vi "MODEL SELECTION.vi"(8 "error in (no error)":errorcluster, 11 "Plan List":string[](array[string])) -> (0 "error out 2":errorcluster, 2 "SELECTED RECIPE\nand COMBI OF BIN- INDEX":cluster{"RECIPE INDEX":i32, "COMBI BIN":i32}, 3 "Plan Selected":string(combo))   [LabVIEW 2017]
panel:
  in  "RECIPE SELECT":string(combo)
  in  "Cancel Button":bool
  in  "Save Button":bool
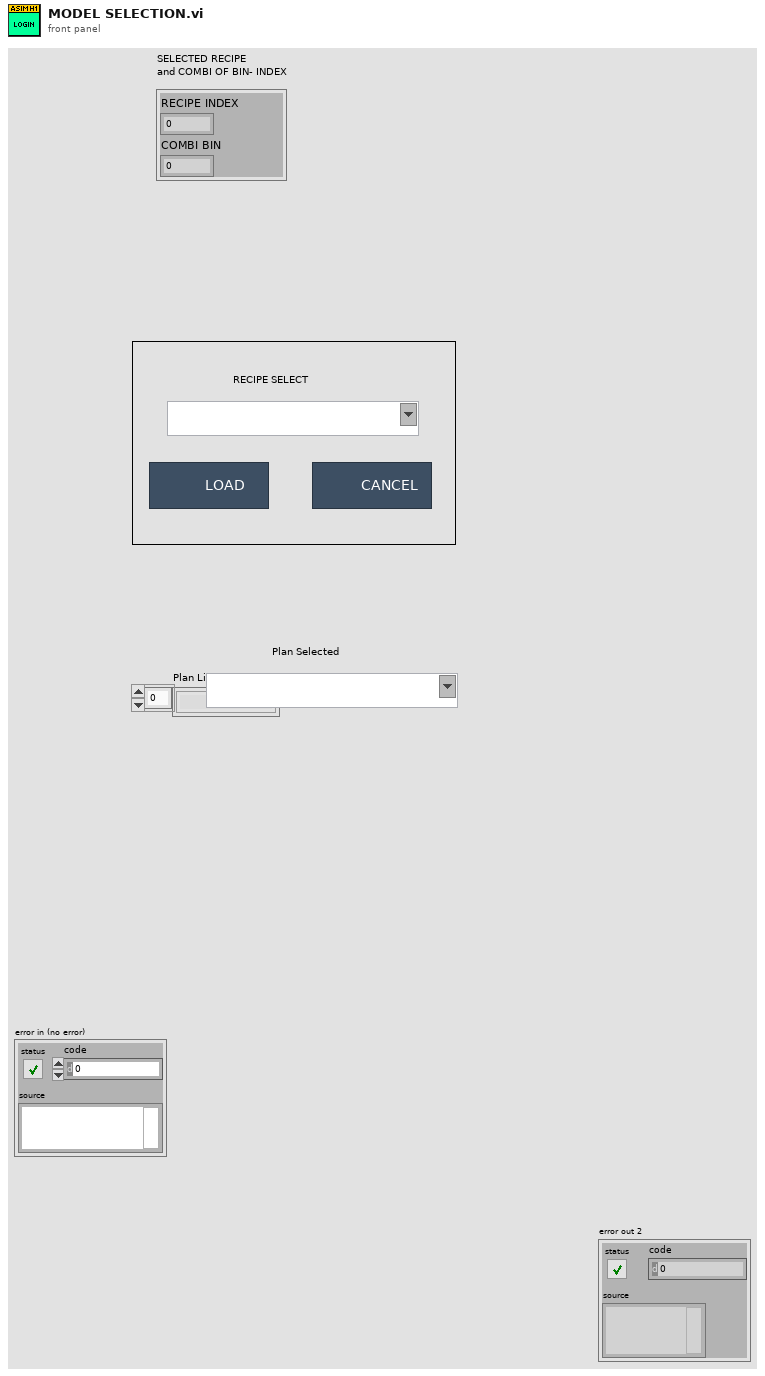
[diagram p1: front panel]
types:
  T1 = enum32{"invalid app kind", "Development System", "Run Time System", "Student Edition", "Embedded LabVIEW", "Evaluation", "Custom"}
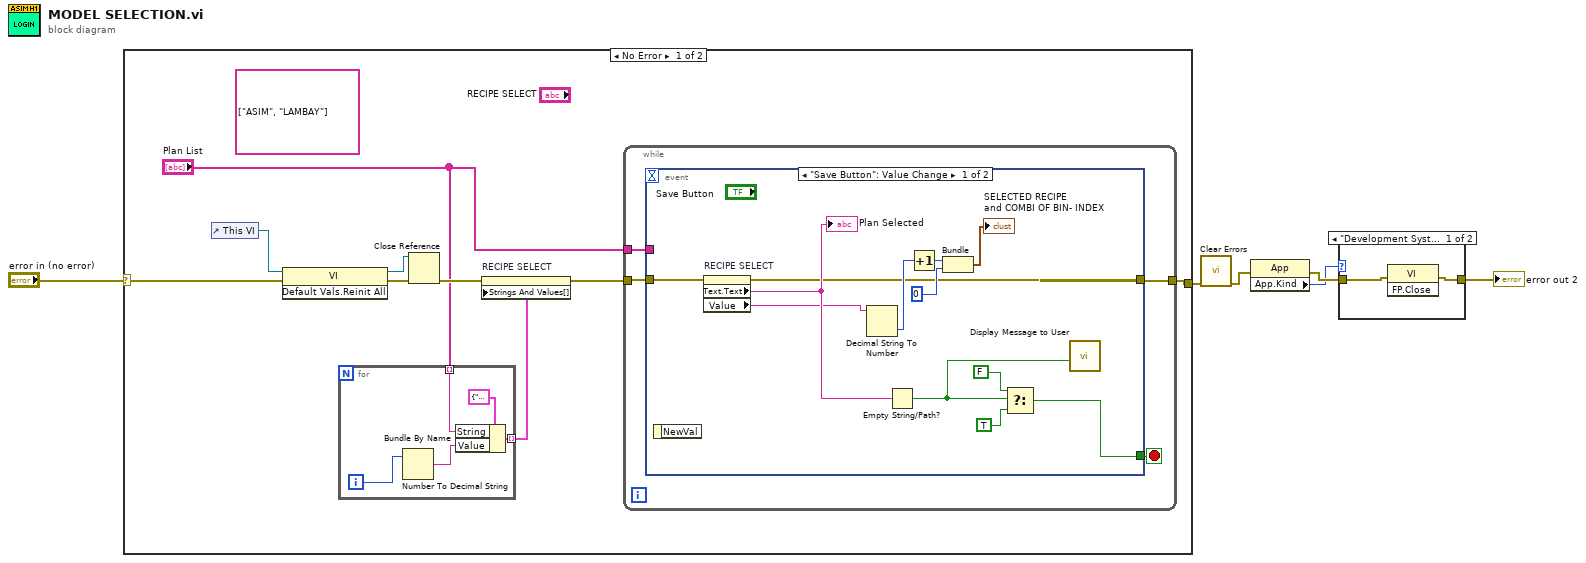
[diagram p0: block diagram]
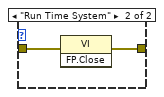
[diagram p2: hidden frame]
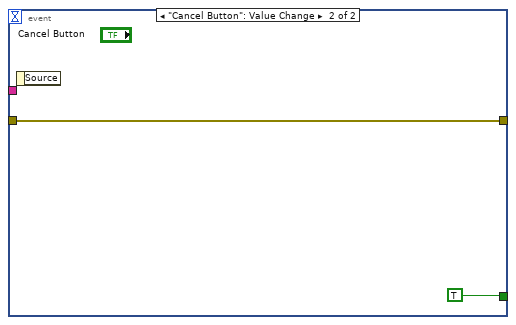
[diagram p3: hidden frame]
diagram:
  n1 = case shown="No Error" "error in (no error)" {
    selector: "error in (no error)" -> [w13 w39]
    tunnel: [w15 w39] -> w6
    frame No Error {
      (unwired) string[] ["ASIM", "LAMBAY"]
      n2 = control-ref of="This VI"() -> (w14:refnum<vi>)
      n3 = invoke class="VI" method="Default Vals.Reinit All"(reference=w14, error in=w13) -> (reference out=w12:refnum<vi>, error out=w11:errorcluster)  [unwired: 1 in, 1 out]
      n4 = for {
        tunnel: "Plan List" -> [w17] mode=indexing
        tunnel: [w16] -> w8 mode=indexing
        i -> [w19]
        n5 = Number To Decimal String(number=w19) -> (decimal integer string=w18:string)  [unwired: 1 in]
        n6 = Bundle By Name(cluster=cluster{"String":string, "Value":string} {"String"="", "Value"=""}, "String"=w17, "Value"=w18) -> (w16:cluster{"String":string, "Value":string})
      }
      n7 = Close Reference(reference=w12, error in (no error)=w11) -> (error out=w9:errorcluster)
      n8 = property on="RECIPE SELECT" class="CmbBox"(error in=w9, "Strings And Values[]"=w8) -> (error out=w10:errorcluster)  [unwired: 1 in, 1 out]
      n9 = while {
        tunnel: w10 -> [w22]
        tunnel: [w23] -> w15
        tunnel: "Plan List" -> [w21]
        stop <- w24 stop-if-true
        n10 = event shown="[0] \"Save Button\": Value Change" {
          selector: _ -> [_ _]
          dyn-events: _ -> [_ _]
          timeout: _ -> [_ _]
          tunnel: [w34 TRUE] -> w24
          tunnel: [w25 w37] -> w23
          tunnel: w22 -> [w26 w37]
          tunnel: w21 -> [_ _]
          event "Save Button": Value Change {
            n11 = event-data() -> ()  [unwired: 1 in, 1 out]
            n12 = property on="RECIPE SELECT" class="CmbBox"(error in=w26) -> (error out=w25:errorcluster, "Text.Text"=w29:string, "Value"=w28:string)  [unwired: 1 in, 1 out]
            "Plan Selected" <- w29
            n13 = Decimal String To Number(string=w28) -> (number=w27:i32)  [unwired: 2 in, 1 out]
            n14 = Empty String/Path?(string/path=w29) -> (empty?=w33:bool)
            n15 = Increment(x=w27) -> (x+1=w30:i32)
            n16 = Bundle(w30, 0) -> (→"SELECTED RECIPE\nand COMBI OF BIN- INDEX":cluster{i32, i32})  [unwired: 1 in]
            n17 = Select(t=FALSE, s=w33, f=TRUE) -> (s? t:f=w34:bool)
            n18 = call "Display Message to User"("Enable"=w33) -> ()  [unwired: 9 in, 2 out]
          }
          event "Cancel Button": Value Change {
            n19 = event-data() -> ()  [unwired: 1 in, 1 out]
          }
        }
      }
    }
    frame Error {
    }
  }
  n20 = call <vilib>:"Clear Errors.vi"("error in (no error)"=w6) -> ("error out"=w4:errorcluster)  [unwired: 5 in, 1 out]
  n21 = property class="App"(error in=w4) -> (error out=w2:errorcluster, "App.Kind"=w1:T1)  [unwired: 1 in, 1 out]
  n22 = case shown="\"Development System\", Default" w1 {
    tunnel: [w40 w43] -> w3
    tunnel: w2 -> [w41 w42]
    frame "Development System", Default {
      n23 = invoke class="VI" method="FP.Close"(error in=w41) -> (error out=w40:errorcluster)  [unwired: 2 in, 2 out]
    }
    frame "Run Time System" {
      n24 = invoke class="VI" method="FP.Close"(error in=w42) -> (error out=w43:errorcluster)  [unwired: 2 in, 2 out]
    }
  }
  "error out 2" <- w3
